vi "Position_Based_L4_Motion_deg_v2.vi"(9 "Assign z":dbl, 10 "Iris Center":dbl[](array[numeric]), 11 "Tip Position":dbl[](array[numeric])) -> (3 "L4 Motion [deg]":dbl)   [LabVIEW 2016]
doc: "This VI calculates the L4 motion based on the current (x,~,z) position.\nIt is designed so that the aspiration hole is always facing towards a virtual axis (EyeCenter x val,~,assign z)."
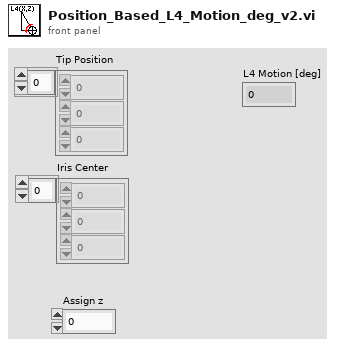
[diagram p1: front panel]
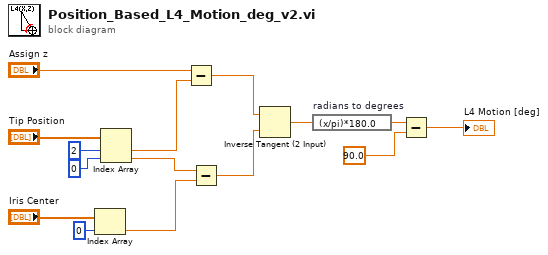
[diagram p0: block diagram]
diagram:
  n1 = Index Array(array="Iris Center", index=0) -> (element=w1:dbl)
  n2 = Index Array(array="Tip Position", index #1=2 ("index"), index #2=0 ("index")) -> (element #1=w6:dbl, element #2=w5:dbl)
  n3 = Subtract(x="Assign z", y=w6) -> (x-y=w14:dbl)
  n4 = Subtract(x=w5, y=w1) -> (x-y=w13:dbl)
  n5 = Inverse Tangent (2 Input)(1:w13, 2:w14) -> (0:w12:dbl)
  n6 = expression code="(x/pi)*180.0" "radians to degrees"(w12) -> (w11:dbl)
  n7 = Subtract(x=w11, y=90.0) -> (x-y=→"L4 Motion [deg]":dbl)
